vi "Waveform Circular Buffer.vi"(8 "error in":errorcluster, 9 "reset":bool, 11 "waveform in":waveform(dbl)[](array[waveform])) -> (0 "error out":errorcluster, 3 "waveform out":waveform(dbl)[](array[waveform]))   [LabVIEW 2019, in "Instrument.Lockin.lvlib" / "Instrument UI.Lockin.lvclass"]
doc: "Circular buffer for the waveform datatype, designed for use with continuous data acquisition. The output is a single waveform with duration <b>buffer duration (s)</b>, in seconds. Input waveforms are appended to the end of the output waveform, and elements older than the buffer duration are discarded.\n\nAll input waveforms must have matching <i>dt</i> values. To eliminate drift in sample times, only the most recent trigger timestamp is considered; the trigger timestamp of the output waveform is computed from the most recently input trigger timestamp, the duration of the buffer, and <i>dt</i>. This may introduce jitter in sample times if the difference between the final timestamp of the previous input and the trigger timestamp of the next input are not exactly equal to <i>dt</i>. In this case, the timestamps of the most recent portion of the buffer will be correct, but earlier timestamps will be scaled. In buffered continuous acquisition, waveforms are consecutive and no jitter is introduced by this method.\n\nThe duration of the buffer may be larger than the requested duration if the duration is not an integer multiple of <i>dt</i>.\n\nOn first call, the input waveform fills end of the buffer; earlier values are set to zero, and the trigger timestamp is backdated. For performance reasons, <b>buffer duration (s)</b> is read only on first call."
uses:
  Instrument UI.Lockin.lvclass
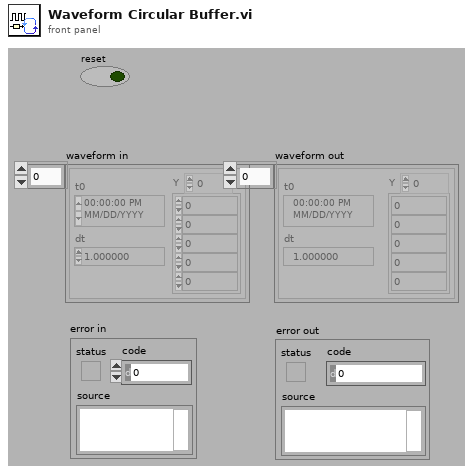
[diagram p1: front panel]
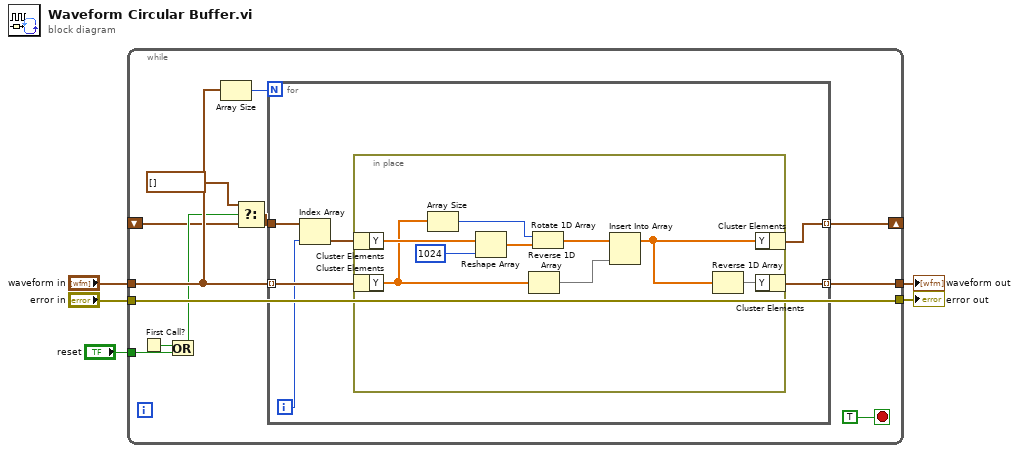
[diagram p0: block diagram]
diagram:
  n1 = while {
    tunnel: "waveform in" -> [w13]
    tunnel: [w17] -> w4
    tunnel: "error in" -> [w17]
    tunnel: "reset" -> [w15]
    shift-right: [w12] -> _
    shift-left: _ -> [w8]
    tunnel: [w11] -> w1
    stop <- TRUE stop-if-true
    n2 = First Call?() -> (First Call?: T/F=w16:bool)
    n3 = Or(x=w16, y=w15) -> (x .or. y?=w9:bool)
    n4 = Array Size(array=w13) -> (size(s)=w14:i32)
    n5 = Select(t=waveform(dbl)[] [], s=w9, f=w8) -> (s? t:f=w7:waveform(dbl)[])
    n6 = for {
      N: w14 -> [_]
      tunnel: w13 -> [w23] mode=indexing
      tunnel: [w19] -> w12 mode=indexing
      tunnel: w7 -> [w22]
      tunnel: [w18] -> w11 mode=indexing
      i -> [w21]
      n7 = Index Array(array=w22, index=w21) -> (element=w20:waveform(dbl))
      n8 = in-place {
        n9 = in-place-cluster #1(w20) -> ("Y"=w31:dbl[])
        n10 = in-place-cluster #2(w23) -> ("Y"=w28:dbl[])
        n11 = Array Size(array=w28) -> (size(s)=w30:i32)
        n12 = Reshape Array(w31, 1024) -> (w29:dbl[])
        n13 = Reverse 1D Array(array=w28) -> (reversed array=w27:dbl[])
        n14 = Rotate 1D Array(1:w29, 2:w30) -> (0:w26:dbl[])
        n15 = Insert Into Array(array=w26, new element=w27) -> (w25:dbl[])  [unwired: 1 in]
        n16 = Reverse 1D Array(array=w25) -> (reversed array=w24:dbl[])
        n17 = in-place-cluster #1("Y"=w25) -> (w19:waveform(dbl))
        n18 = in-place-cluster #2("Y"=w24) -> (w18:waveform(dbl))
      }
    }
  }
  "waveform out" <- w1
  "error out" <- w4
